vi "Line Detector Interpolate Signal.vi"(7 "Frequency":dbl[](array[numeric]), 9 "Signal Y":dbl[](array[numeric]), 10 "Signal X":dbl[](array[numeric]), 11 "Spectrum Recorder Configuration":T1={"Start frequency"=500000.0, "End frequency"=2000000.0, "Frequency step"=100.0, "Step duration"=0.004, "Red Pitaya address"="192.168.1.100", "Open plot \non start"=FALSE, "Focus region centers"=[], "Regions width"=2000.0, "Out-of-focus\nstep acceleration"=1} {"Out-of-focus\nstep acceleration" min=1; "Regions width" format="%#_6pHz"; "Focus region centers" format="%#_6pHz"; "Step duration" format="%#_6ps"; "Frequency step" format="%#_6pHz"; "End frequency" format="%#_6pHz"; "Start frequency" format="%#_6pHz"}) -> (1 "Signal Y out":dbl[](array[numeric]), 2 "Signal X out":dbl[](array[numeric]), 3 "Steps":dbl[](array[numeric]) format="%#_8p", 5 "Frequency out":dbl[](array[numeric]))   [LabVIEW 2016]
uses:
  Red Pitaya/RP Core/Red Pitaya Transceiver Driver/Spectrum Configuration.ctl
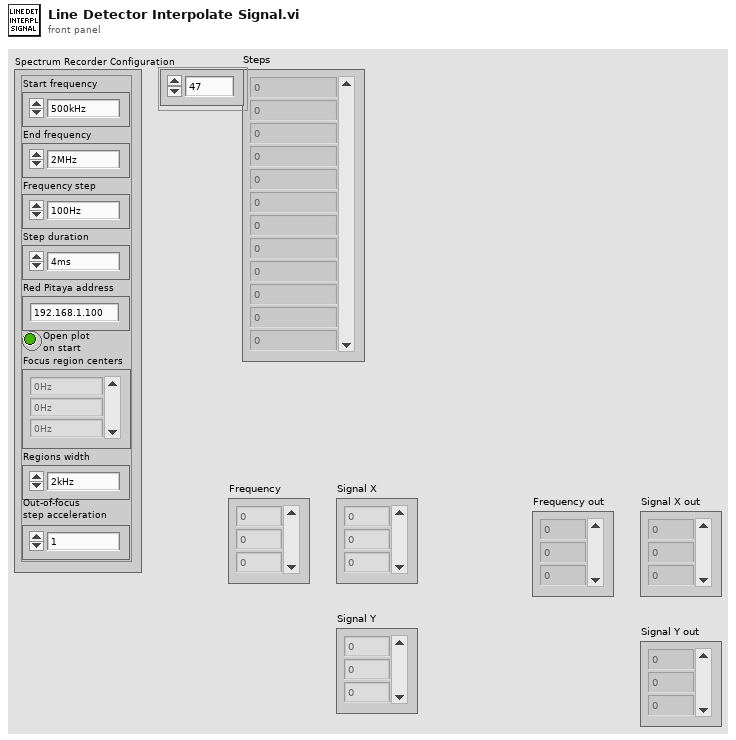
[diagram p1: front panel]
types:
  T1 = typedef "Spectrum Configuration.ctl" = cluster{"Start frequency":dbl, "End frequency":dbl, "Frequency step":dbl, "Step duration":dbl, "Red Pitaya address":string, "Open plot \non start":bool, "Focus region centers":dbl[], "Regions width":dbl, "Out-of-focus\nstep acceleration":i32}
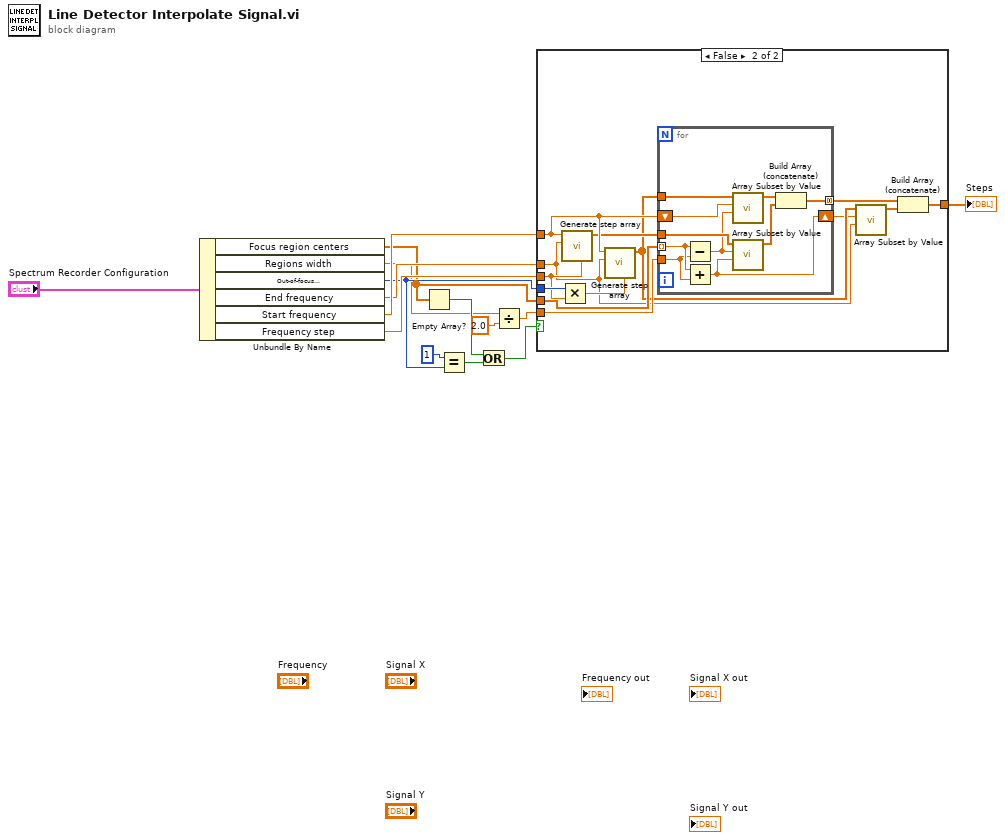
[diagram p0: block diagram]
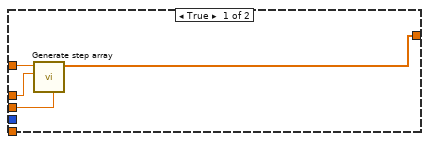
[diagram p2: hidden frame]
diagram:
  n1 = Unbundle By Name("Spectrum Recorder Configuration") -> ("Focus region centers"=w4:dbl[], "Regions width"=w3:dbl, "Out-of-focus\nstep acceleration"=w5:i32, "End frequency"=w12:dbl, "Start frequency"=w13:dbl, "Frequency step"=w14:dbl)
  n2 = Empty Array?(array=w4) -> (empty?=w7:bool)
  n3 = Equal?(x=1, y=w5) -> (x = y?=w8:bool)
  n4 = Or(x=w7, y=w8) -> (x .or. y?=w6:bool)
  n5 = Divide(x=w3, y=2.0) -> (x/y=w1:dbl)
  n6 = case shown="False" w6 {
    tunnel: [w15 w19] -> w10
    tunnel: w12 -> [w17 w22]
    tunnel: w13 -> [w18 w26]
    tunnel: w14 -> [w16 w30]
    tunnel: w5 -> [_ w31]
    tunnel: w4 -> [_ w28]
    tunnel: w1 -> [_ w27]
    frame True {
      n7 = call "Generate step array.vi"("Step"=w16, "End"=w17, "Start"=w18) -> ("Steps"=w15:dbl[])  [unwired: 8 in]
    }
    frame False {
      n8 = Multiply(x=w31, y=w30) -> (x*y=w29:dbl)
      n9 = call "Generate step array.vi"("Step"=w30, "End"=w22, "Start"=w26) -> ("Steps"=w25:dbl[])  [unwired: 8 in]
      n10 = call "Generate step array.vi"("Step"=w29, "End"=w22, "Start"=w26) -> ("Steps"=w24:dbl[])  [unwired: 8 in]
      n11 = for {
        tunnel: w28 -> [w37] mode=indexing
        tunnel: w24 -> [w41]
        tunnel: w27 -> [w36]
        shift-right: [w32] -> w23
        shift-left: w26 -> [w40]
        tunnel: w25 -> [w39]
        tunnel: [w33] -> w21 mode=concatenating
        n12 = Subtract(x=w37, y=w36) -> (x-y=w38:dbl)
        n13 = Add(x=w37, y=w36) -> (x+y=w32:dbl)
        n14 = call "Array Subset by Value.vi"("End"=w38, "Start"=w40, "Data"=w41) -> ("Data subset"=w35:dbl[])  [unwired: 8 in]
        n15 = call "Array Subset by Value.vi"("End"=w32, "Start"=w38, "Data"=w39) -> ("Data subset"=w34:dbl[])  [unwired: 8 in]
        n16 = Build Array (concatenate)(w35, w34) -> (w33:dbl[])
      }
      n17 = call "Array Subset by Value.vi"("End"=w22, "Start"=w23, "Data"=w24) -> ("Data subset"=w20:dbl[])  [unwired: 8 in]
      n18 = Build Array (concatenate)(w21, w20) -> (w19:dbl[])
    }
  }
  "Steps" <- w10
